vi "报警XML解析.vi"(8 "error in (no error)":errorcluster caption="错误输入（无错误）", 11 "筛选输入":T1={"componentParent"="斯坦道营养盐", "componentName"="", "equipVersion"="B", "Code"=""}) -> (0 "error out":errorcluster caption="错误输出", 3 "data":T2(array[cluster]))   [LabVIEW 2016, in "Alarm interface.lvlib"]
uses:
  Alarm interface.lvlib
  <vilib>/xml/Load XML File.vi
  <vilib>/xml/Close Reference(Node).vi
  <vilib>/xml/NI_XML.lvlib
  <resource>/objmgr/DOMUserDefRef.rc
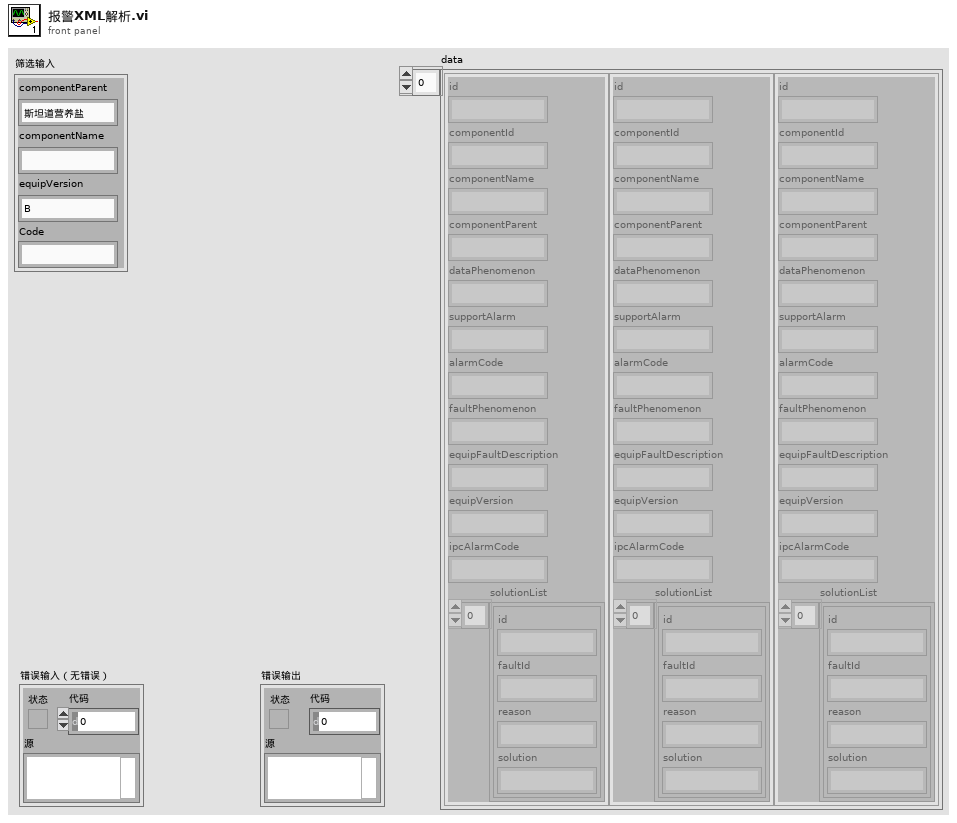
[diagram p1: front panel]
types:
  T1 = cluster{"componentParent":string, "componentName":string, "equipVersion":string, "Code":string}
  T2 = cluster{"id":string, "componentId":string, "componentName":string, "componentParent":string, "dataPhenomenon":string, "supportAlarm":string, "alarmCode":string, "faultPhenomenon":string, "equipFaultDescription":string, "equipVersion":string, "ipcAlarmCode":string, "solutionList":cluster{"id":string, "faultId":string, "reason":string, "solution":string}[]}[]
  T3 = cluster{"node text":string, "node text":string, "node text":string, "node text":string}
  T4 = cluster{"id":string, "componentId":string, "componentName":string, "componentParent":string, "dataPhenomenon":string, "supportAlarm":string, "alarmCode":string, "faultPhenomenon":string, "equipFaultDescription":string, "equipVersion":string, "ipcAlarmCode":string, "solutionList":cluster{"id":string, "faultId":string, "reason":string, "solution":string}[]}
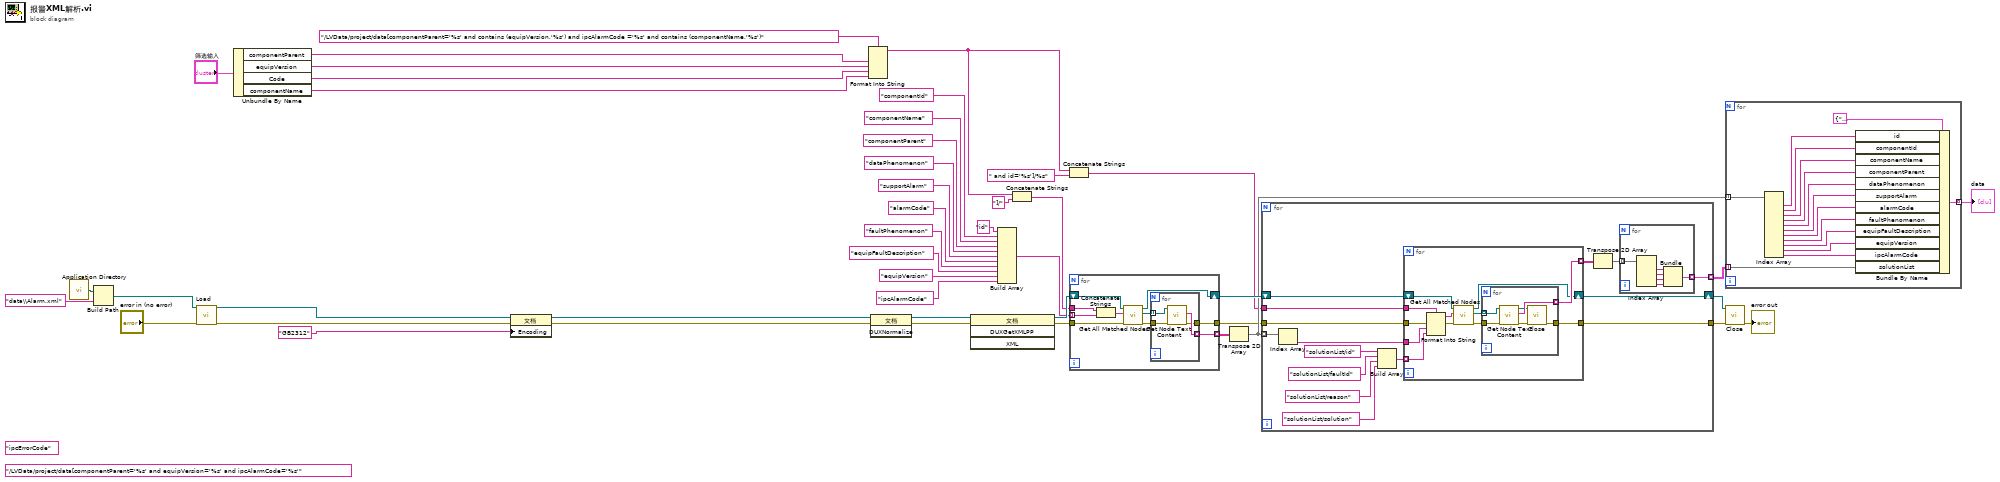
[diagram p0: block diagram]
diagram:
  (unwired) "/LVData/project/data[componentParent='%s' and equipVersion='%s' and ipcAlarmCode='%s'" ("格式字符串")
  (unwired) "ipcErrorCode"
  n1 = call <vilib>:"Application Directory.vi"() -> ("Application Directory"=w9:path)
  n2 = Build Path(base path=w9, name or relative path="data\\Alarm.xml" ("字符串")) -> (appended path=w7:path)
  n3 = call-poly <vilib>:"Load.vi"("path to XML document"=w7, "error in (no error)"="error in (no error)") -> ("DOM document out"=w42:refnum<k20>, "error out"=w41:errorcluster)  [unwired: 11 in, 1 out]
  n4 = Unbundle By Name("筛选输入") -> ("componentParent"=w10:string, "equipVersion"=w3:string, "Code"=w4:string, "componentName"=w1:string)
  n5 = property on="属性节点" class="文档"(reference=w42, error in=w41, "Encoding"="GB2312" ("文档编码")) -> (reference out=w44:refnum<k20>, error out=w43:errorcluster)
  n6 = Format Into String(format string="/LVData/project/data[componentParent='%s' and contains (equipVersion,'%s') and ipcAlarmCode ='%s' and contains (componentName,'%s')" ("字符串"), w10, w3, w4, w1) -> (resulting string=w6:string)  [unwired: 2 in, 1 out]
  n7 = invoke on="调用节点" class="文档" method="DUXNormalize"(reference=w44, error in=w43) -> (reference out=w40:refnum<k20>, error out=w39:errorcluster)  [unwired: 1 in, 1 out]
  n8 = invoke on="调用节点" class="文档" method="DUXGetXMLPP"(reference=w40, error in=w39) -> (reference out=w28:refnum<k20>, error out=w14:errorcluster)  [unwired: 2 in, 2 out]
  n9 = Build Array("id", "componentId", "componentName", "componentParent", "dataPhenomenon", "supportAlarm", "alarmCode", "faultPhenomenon", "equipFaultDescription", "equipVersion", "ipcAlarmCode") -> (w27:string[])
  n10 = Concatenate Strings(w6, "]/" ("字符串")) -> (w19:string)
  n11 = Concatenate Strings(w6, " and id='%s']/%s" ("字符串")) -> (w17:string)
  n12 = for {
    tunnel: w19 -> [w49]
    tunnel: w27 -> [w48] mode=indexing
    tunnel: [w53] -> w26 mode=indexing
    tunnel: [w50] -> w15
    tunnel: w14 -> [w47]
    shift-right: [w52] -> w25
    shift-left: w28 -> [w55]
    n13 = Concatenate Strings(w49, w48) -> (w46:string)
    n14 = call <vilib>:"Get All Matched Nodes.vi"("error in (no error)"=w47, "XPath expression"=w46, "node in"=w55) -> ("error out"=w51:errorcluster, "node result array"=w54:refnum<k20>[], "node out"=w52:refnum<k20>)  [unwired: 6 in]
    n15 = for {
      tunnel: w54 -> [w59] mode=indexing
      tunnel: [w58] -> w53 mode=indexing
      tunnel: w51 -> [w57]
      tunnel: [w56] -> w50
      n16 = call <vilib>:"Get Node Text Content.vi"("error in (no error)"=w57, "node in"=w59) -> ("error out"=w56:errorcluster, "node text"=w58:string)  [unwired: 7 in, 1 out]
    }
  }
  n17 = Transpose 2D Array(2D array=w26) -> (transposed array=w22:string[][])
  n18 = for {
    tunnel: w22 -> [w74] mode=indexing
    tunnel: w17 -> [w73]
    tunnel: [w62] -> w23 mode=indexing
    tunnel: w15 -> [w61]
    tunnel: [w60] -> w13
    shift-right: [w64] -> w24
    shift-left: w25 -> [w71]
    n19 = Index Array(array=w74) -> (element=w72:string)  [unwired: 1 in]
    n20 = Build Array("solutionList/id" ("XPath expression"), "solutionList/faultId" ("XPath expression"), "solutionList/reason" ("XPath expression"), "solutionList/solution" ("XPath expression")) -> (w66:string[])
    n21 = for {
      tunnel: w73 -> [w92]
      tunnel: w72 -> [w91]
      tunnel: w66 -> [w90] mode=indexing
      tunnel: [w86] -> w65 mode=indexing
      tunnel: w61 -> [w84]
      tunnel: [w81] -> w60
      shift-right: [w85] -> w64
      shift-left: w71 -> [w88]
      n22 = Format Into String(format string=w92, error in=w84, w91, w90) -> (resulting string=w87:string, error out=w83:errorcluster)  [unwired: 1 in]
      n23 = call <vilib>:"Get All Matched Nodes.vi"("error in (no error)"=w83, "XPath expression"=w87, "node in"=w88) -> ("error out"=w82:errorcluster, "node result array"=w89:refnum<k20>[], "node out"=w85:refnum<k20>)  [unwired: 6 in]
      n24 = for {
        tunnel: w89 -> [w98] mode=indexing
        tunnel: [w97] -> w86 mode=indexing
        tunnel: w82 -> [w96]
        tunnel: [w93] -> w81
        n25 = call <vilib>:"Get Node Text Content.vi"("error in (no error)"=w96, "node in"=w98) -> ("error out"=w94:errorcluster, "node text"=w97:string, "node out"=w95:refnum<k20>)  [unwired: 7 in]
        n26 = call-poly <vilib>:"Close.vi"("error in (no error)"=w94, "node"=w95) -> ("error out"=w93:errorcluster)  [unwired: 7 out]
      }
    }
    n27 = Transpose 2D Array(2D array=w65) -> (transposed array=w63:string[][])
    n28 = for {
      tunnel: w63 -> [w80] mode=indexing
      tunnel: [w75] -> w62 mode=indexing
      n29 = Index Array(array=w80) -> (element #1=w79:string, element #2=w78:string, element #3=w77:string, element #4=w76:string)  [unwired: 4 in]
      n30 = Bundle("node text"=w79, "node text"=w78, "node text"=w77, "node text"=w76) -> (w75:T3)  [unwired: 1 in]
    }
  }
  n31 = for {
    tunnel: w22 -> [w103] mode=indexing
    tunnel: [w104] -> w21 mode=indexing
    tunnel: w23 -> [w102] mode=indexing
    n32 = Index Array(array=w103) -> (element #1=w112:string, element #2=w111:string, element #3=w110:string, element #4=w109:string, element #5=w108:string, element #6=w107:string, element #7=w100:string, element #8=w106:string, element #9=w105:string, element #10=w101:string, element #11=w99:string)  [unwired: 11 in]
    n33 = Bundle By Name(cluster=T4 {"id"="", "componentId"="", "componentName"="", "componentParent"="", "dataPhenomenon"="", "supportAlarm"="", "alarmCode"="", "faultPhenomenon"="", "equipFaultDescription"="", "equipVersion"="", "ipcAlarmCode"="", "solutionList"=[]} ("data"), "id"=w112, "componentId"=w111, "componentName"=w110, "componentParent"=w109, "dataPhenomenon"=w108, "supportAlarm"=w107, "alarmCode"=w100, "faultPhenomenon"=w106, "equipFaultDescription"=w105, "equipVersion"=w101, "ipcAlarmCode"=w99, "solutionList"=w102) -> (w104:T4)
  }
  "data" <- w21
  n34 = call-poly <vilib>:"Close.vi"("error in (no error)"=w13, "node"=w24) -> ("error out"=→"error out":errorcluster)  [unwired: 7 out]
